vi "test02.vi"() -> ()   [LabVIEW 2019]
uses:
  <userlib>/KNR OS 4.0 LabVIEW Toolkit/F710/f710.ctl
  <vilib>/Platform/TimedLoop/XDataNode/timing_clust.ctl
  <vilib>/Platform/TimedLoop/XDataNode/nitl_modes.ctl
  <vilib>/Platform/TimedLoop/XDataNode/wakeup.ctl
  <vilib>/platform/TimedLoop/XDataNode/XDataNode.xnode
  <vilib>/Platform/TimedLoop/XDataNode/XDNodeRunTimeDep.lvlib
panel:
  out "error out 2":errorcluster
  out "F710":T1
  in  "stop":bool
  out "error out":errorcluster
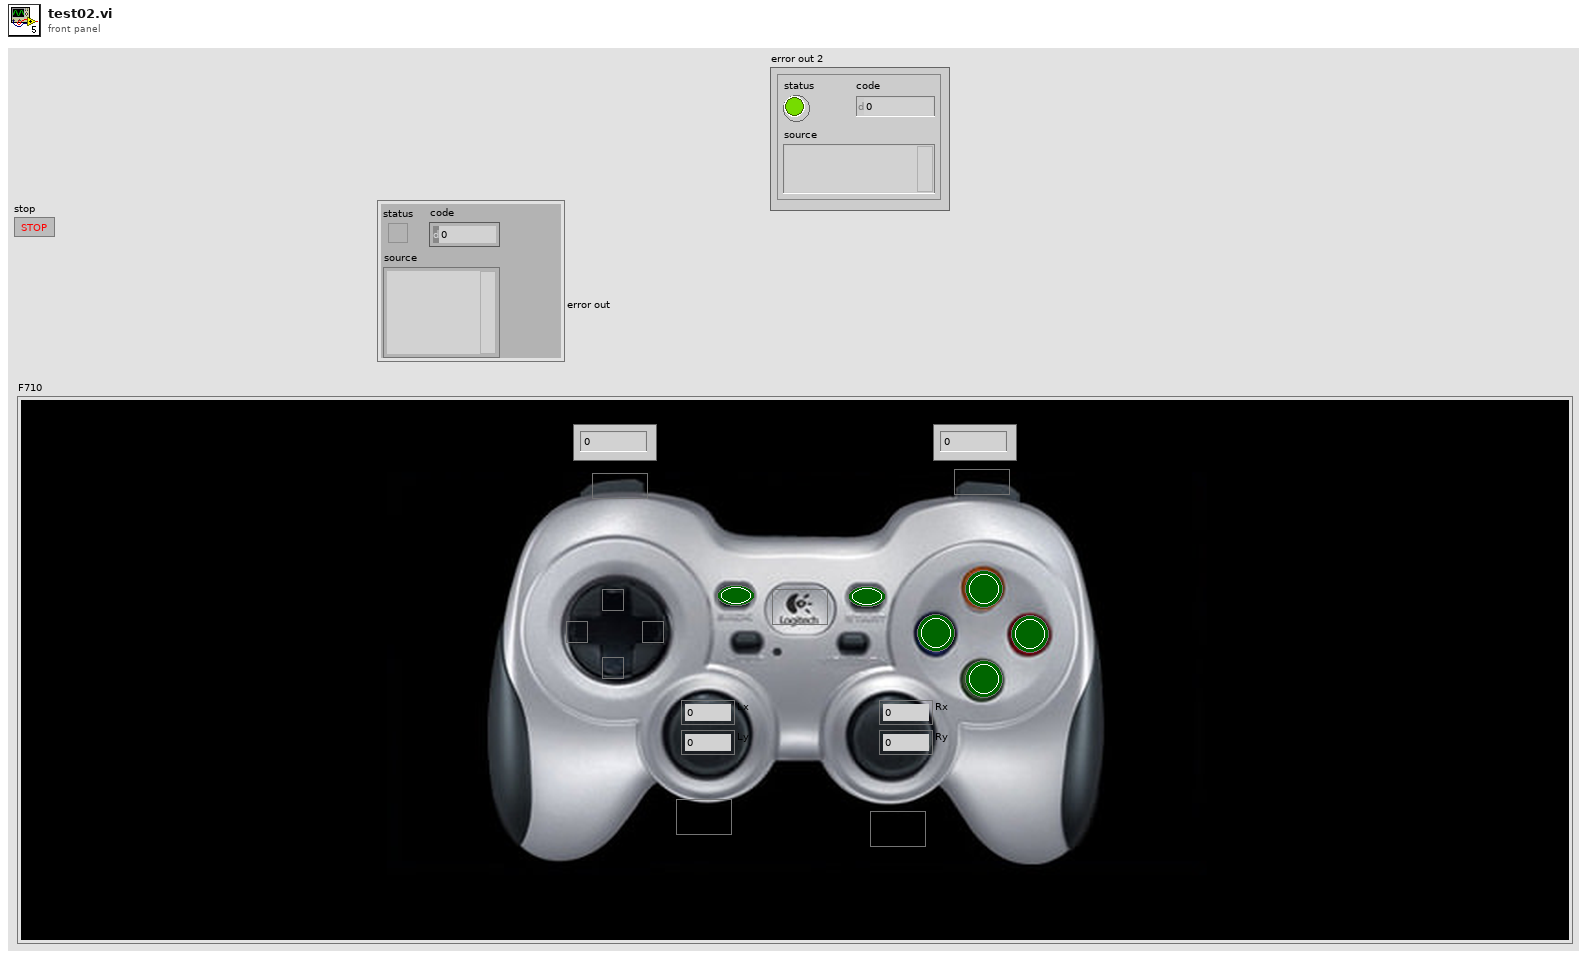
[diagram p1: front panel]
types:
  T1 = typedef "f710.ctl" = cluster{"Down":bool, "Left":bool, "Up":bool, "Right":bool, "A":bool, "X":bool, "Y":bool, "B":bool, "LB":bool, "RB":bool, "LT":i16, "RT":i16, "L3":bool, "R3":bool, "Ly":i16, "Lx":i16, "Ry":i16, "Rx":i16, "Back":bool, "Start":bool, "center":bool}
  T2 = typedef "XDNodeRunTimeDep.lvlib/timing_clust.ctl" = cluster{"Expected End [f-1]":u64, "Actual End [f-1]":u64, "Finished Late? [f-1]":bool, "Expected End [i-1]":u64, "Actual End [i-1]":u64, "Finished Late? [i-1]":bool, "Expected Start [i]":u64, "Actual Start [i]":u64, "Expected Start [f]":u64, "Actual Start [f]":u64, "Source Name":string, "Structure Name":string, "Period":i64, "Deadline":i64, "Offset":i64, "Start":i64, "Priority":i32, "Timeout":i32, "Mode":T3, "Wakeup Reason":T4, "Error":errorcluster, "Source Type":string, "Secondary Source Type":string, "Global End Time":u64, "Global Start Time":u64, "Frame Duration":u64, "Iteration Duration":u64, "Assigned CPU":i32, "I/O Scan Engine Mode":u32}
  T3 = typedef "XDNodeRunTimeDep.lvlib/nitl_modes.ctl" = enum32{"No Change", "Process missed periods, maintain original phase", "Discard missed periods, maintain original phase", "Process missed periods, ignore original phase", "Discard missed periods, ignore original phase"}
  T4 = typedef "XDNodeRunTimeDep.lvlib/wakeup.ctl" = enum32{"Normal", "Aborted", "Asynchronous wakeup", "Timing source error", "Timed loop error", "Timeout"}
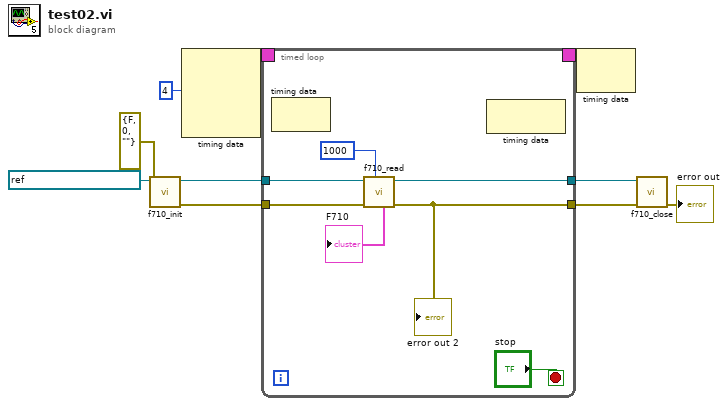
[diagram p0: block diagram]
diagram:
  n1 = call <userlib>:"f710_init.vi"("error in (no error)"=errorcluster {"status"=FALSE, "code"=0, "source"=""}, "USB RAW VISA resource name"=refnum<visa-resource-name> "USB0::0x046D::0xC21F::D637907D::RAW") -> ("error out"=w8:errorcluster, "VISA Refnum out"=w7:refnum<visa-resource-name>)  [unwired: 8 in]
  n2 = node-c288(i64 4 ("Period")) -> (w10:T2)  [unwired: 3 in]
  n3 = timed-loop {
    timing: w10 -> [_]
    timing-out: [_] -> w9
    tunnel: w8 -> [w17]
    tunnel: w7 -> [w16]
    tunnel: [w15] -> w6
    tunnel: [w14] -> w5
    stop <- "stop" stop-if-true
    n4 = node-c288() -> ()  [unwired: 1 in, 1 out]
    n5 = call <userlib>:"f710_read.vi"("Timeout to wait for Interrupt (ms)"=u32 1000, "error in (no error)"=w17, "VISA Refnum in"=w16) -> ("error out"=w14:errorcluster, "VISA Refnum out"=w15:refnum<visa-resource-name>, "F710"=→"F710":T1)  [unwired: 6 in]
    "error out 2" <- w14
    n6 = node-c288() -> ()  [unwired: 1 in, 1 out]
  }
  n7 = node-c288(w9) -> ()  [unwired: 1 out]
  n8 = call <userlib>:"f710_close.vi"("error in (no error)"=w5, "VISA Refnum in"=w6) -> ("error out"=→"error out":errorcluster)  [unwired: 9 in]
